vi "Spectral Data Organize TDMS (SubVI).vi"(0 "Measurement Cluster IN":T2, 1 "Data Array IN":dbl[](array[numeric]), 2 "tdms file":refnum<k34>, 3 "error in (no error)":errorcluster, 5 "Shutter":bool, 7 "Ref Lamp Mode":T1(radio), 9 "Collect Background":bool, 10 "Ref Lamp at Flame Loc File":path=path "C:/Users/bedickc/Documents/_MHD/K Spectroscopy (Ocean Optics Spectrometer)/20171005_HR4000_KOptics_Calib/Lamp_At_Flame_Location_ND10Corr_HR4000_LabviewWavelengths.csv", 11 "Take Ref Lamp":bool, 13 "Integration Time (ms)":dbl format="%#_13g", 14 "ON/OFF IN":bool) -> (4 "Measurement Cluster OUT":T2, 6 "tdms file out":refnum<k34>, 8 "error out":errorcluster)   [LabVIEW 2018]
uses:
  Measurement Cluster.ctl
panel:
  in  "Iteration Number":i32
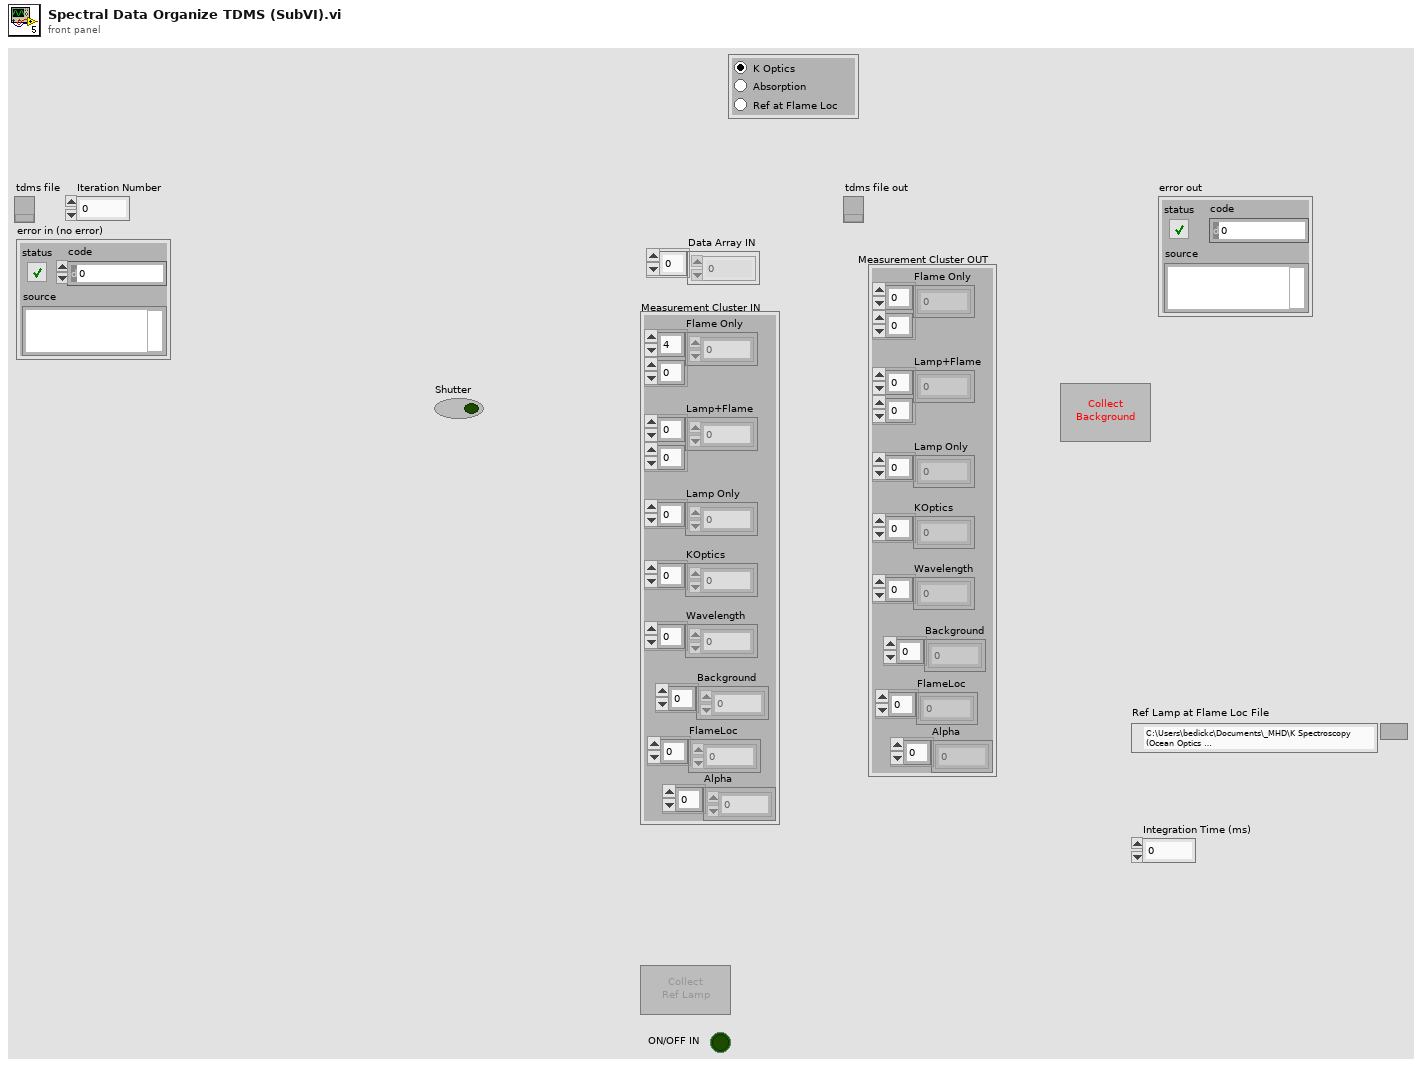
[diagram p1: front panel]
types:
  T1 = enum32{"K Optics", "Absorption", "Ref at Flame Loc"}
  T2 = typedef "Measurement Cluster.ctl" = cluster{"Flame Only":dbl[][], "Lamp+Flame":dbl[][], "Lamp Only":dbl[], "KOptics":dbl[], "Wavelength":dbl[], "Background":dbl[], "FlameLoc":dbl[], "Alpha":dbl[]}
  T3 = enum16{"open", "open or create", "create or replace", "create", "open (read-only)"}
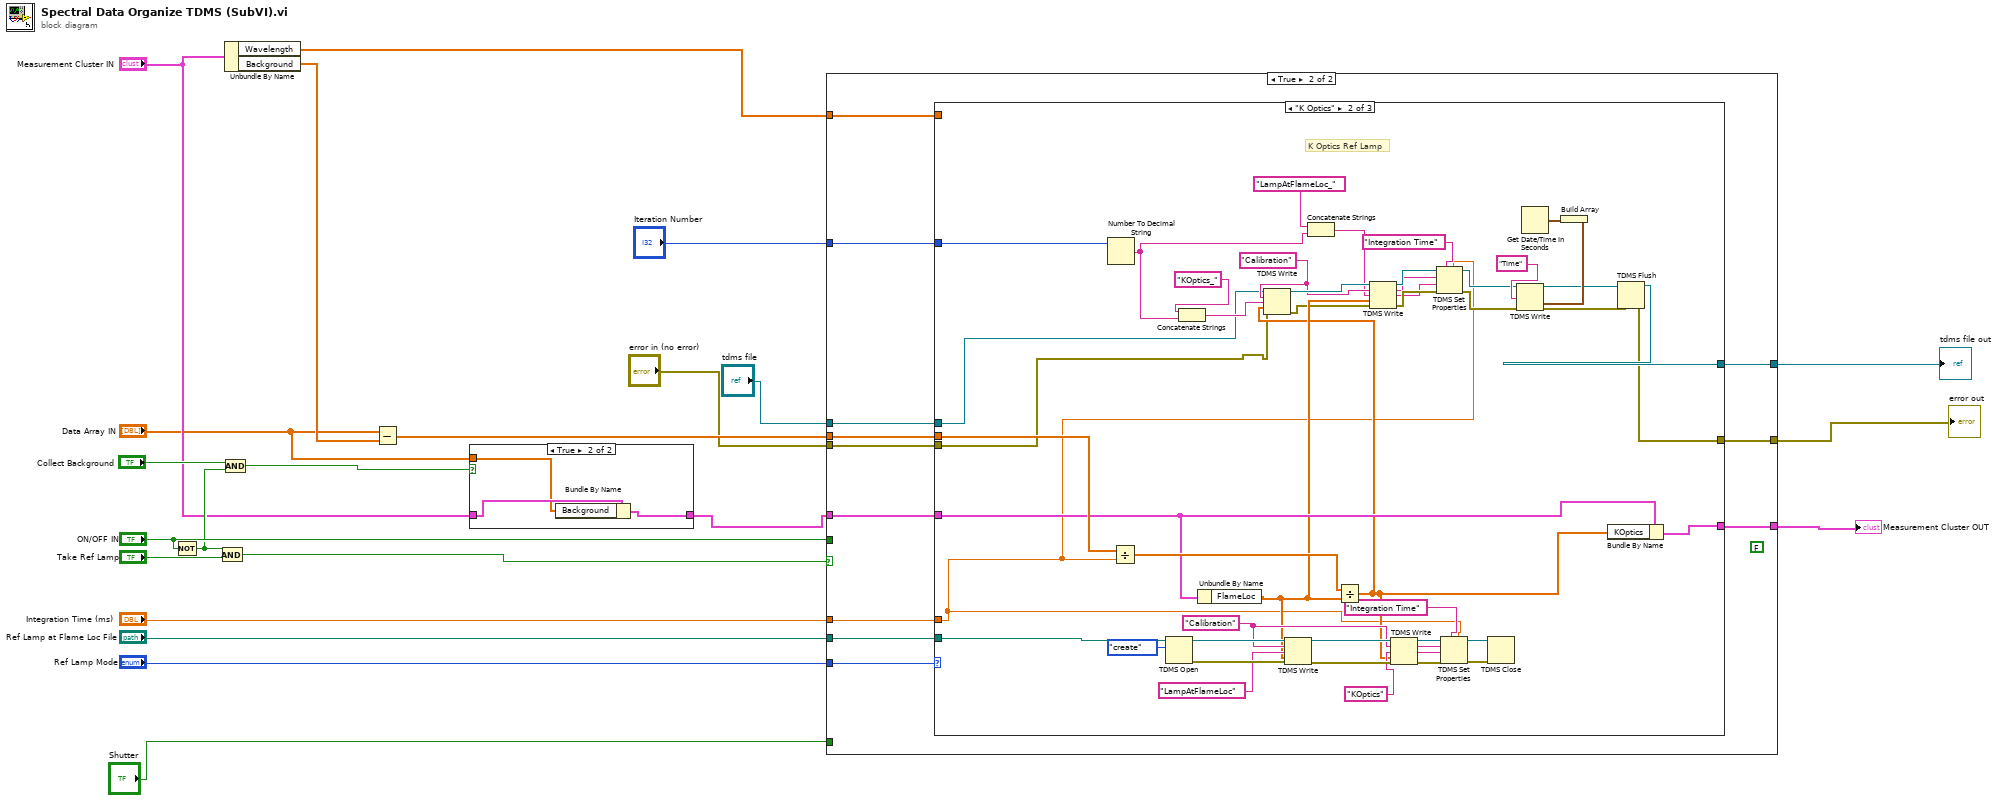
[diagram p0: block diagram]
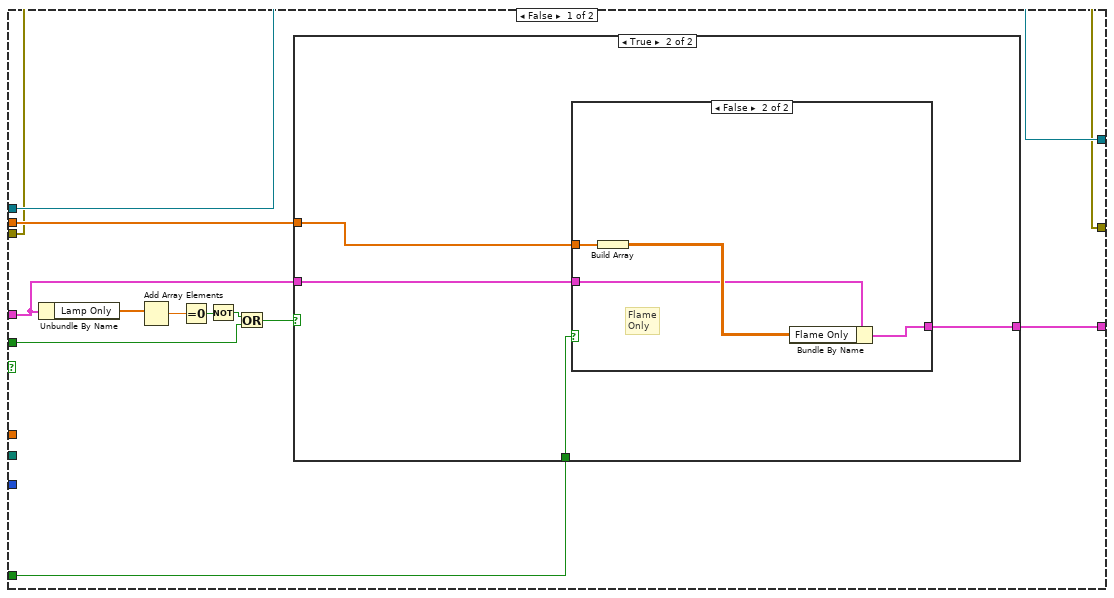
[diagram p2: hidden frame]
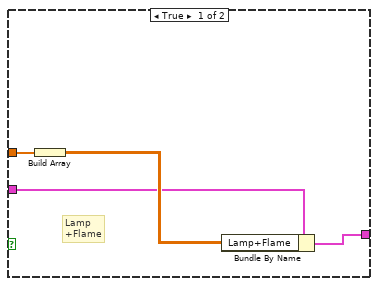
[diagram p4: hidden frame]
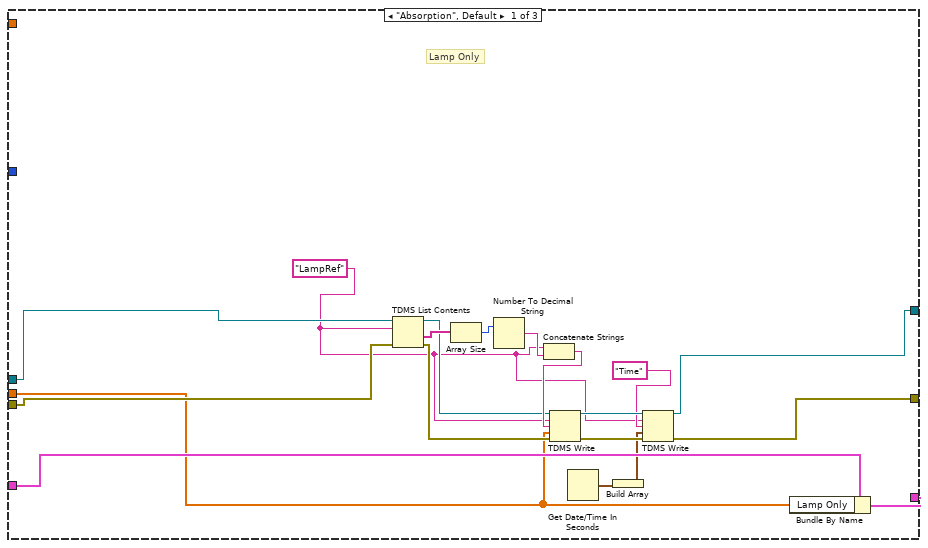
[diagram p5: hidden frame]
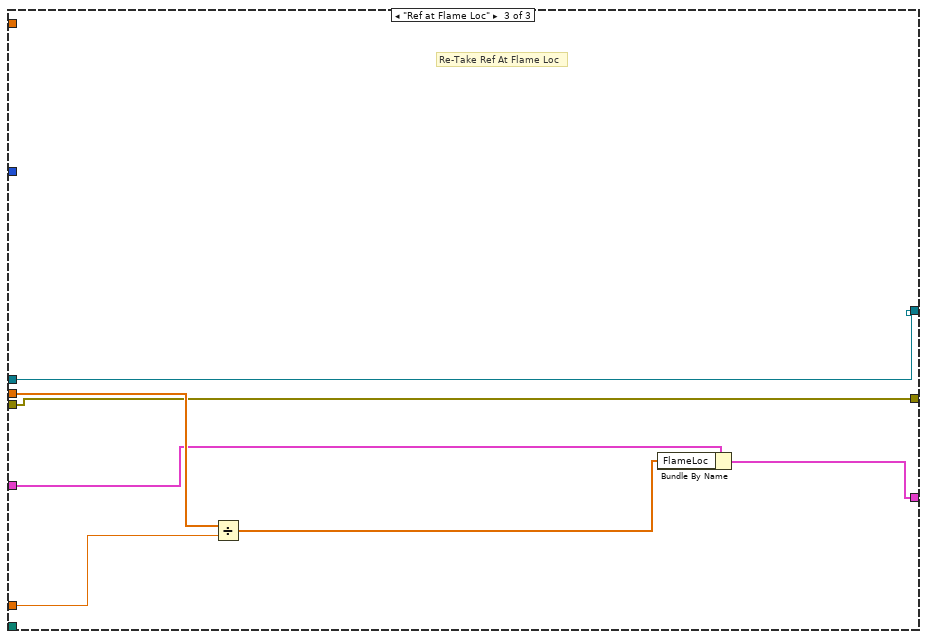
[diagram p6: hidden frame]
diagram:
  n1 = Not(x="ON/OFF IN") -> (.not. x?=w12:bool)
  n2 = Compound Arithmetic op=AND(w12, "Take Ref Lamp") -> (w21:bool)
  n3 = Unbundle By Name("Measurement Cluster IN") -> ("Wavelength"=w19:dbl[], "Background"=w15:dbl[])
  n4 = Compound Arithmetic op=AND("Collect Background", w12) -> (w10:bool)
  n5 = Subtract(x="Data Array IN", y=w15) -> (x-y=w16:dbl[])
  n6 = case shown="True" w10 {
    tunnel: "Measurement Cluster IN" -> [w23 w25]
    tunnel: [w23 w26] -> w6
    tunnel: "Data Array IN" -> [_ w24]
    frame False {
    }
    frame True {
      n7 = Bundle By Name(cluster=w25, "Background"=w24) -> (w26:T2)
    }
  }
  n8 = case shown="True" w21 {
    tunnel: w16 -> [w38 w58]
    tunnel: "ON/OFF IN" -> [w37 _]
    tunnel: "Ref Lamp at Flame Loc File" -> [_ w63]
    tunnel: "Integration Time (ms)" -> [_ w62]
    tunnel: w19 -> [_ w61]
    tunnel: [w34 w60] -> w18
    tunnel: w6 -> [w35 w59]
    tunnel: "Ref Lamp Mode" -> [_ w57]
    tunnel: "Shutter" -> [w31 _]
    tunnel: "tdms file" -> [w28 w56]
    tunnel: "error in (no error)" -> [w27 w55]
    tunnel: [w28 w54] -> w3
    tunnel: [w27 w53] -> w2
    tunnel: "Iteration Number" -> [_ w52]
    frame False {
      n9 = Unbundle By Name(w35) -> ("Lamp Only"=w32:dbl[])
      n10 = Add Array Elements(numeric array=w32) -> (sum=w33:dbl)
      n11 = Equal To 0?(x=w33) -> (x = 0?=w30:bool)
      n12 = Not(x=w30) -> (.not. x?=w29:bool)
      n13 = Or(x=w29, y=w37) -> (x .or. y?=w36:bool)
      n14 = case shown="True" w36 {
        tunnel: w38 -> [_ w43]
        tunnel: w35 -> [w39 w42]
        tunnel: [w39 w41] -> w34
        tunnel: w31 -> [_ w40]
        frame False {
        }
        frame True {
          n15 = case shown="False" w40 {
            tunnel: w43 -> [w47 w51]
            tunnel: w42 -> [w45 w49]
            tunnel: [w44 w48] -> w41
            frame True {
              # "Lamp\n+Flame"
              n16 = Build Array(w47) -> (w46:dbl[][])
              n17 = Bundle By Name(cluster=w45, "Lamp+Flame"=w46) -> (w44:T2)
            }
            frame False {
              # "Flame\nOnly"
              n18 = Build Array(w51) -> (w50:dbl[][])
              n19 = Bundle By Name(cluster=w49, "Flame Only"=w50) -> (w48:T2)
            }
          }
        }
      }
    }
    frame True {
      (unwired) FALSE
      n20 = case shown="\"K Optics\"" w57 {
        tunnel: w63 -> [_ w126 _]
        tunnel: w62 -> [_ w93 w137]
        tunnel: w61 -> [_ _ _]
        tunnel: [w82 w130 w134] -> w60
        tunnel: w59 -> [w81 w127 w135]
        tunnel: w58 -> [w65 w129 w136]
        tunnel: w56 -> [w69 w87 w132]
        tunnel: w55 -> [w68 w86 w131]
        tunnel: [w64 w89 w132] -> w54
        tunnel: [w67 w88 w131] -> w53
        tunnel: w52 -> [_ w106 _]
        frame "Absorption", Default {
          w66 = "LampRef" ("group name in (Untitled)")
          # "Lamp Only"
          n21 = TDMS List Contents(4:w68, 6:w66, 7:w69) -> (0:w75:errorcluster, 1:w80:string[], 3:w76:refnum<k34>)  [unwired: 1 out]
          n22 = Array Size(array=w80) -> (size(s)=w79:i32)
          n23 = Number To Decimal String(number=w79) -> (decimal integer string=w78:string)  [unwired: 1 in]
          n24 = Concatenate Strings(w66, w78) -> (w77:string)
          n25 = TDMS Write(0:w76, 5:w66, 7:w77, 9:w65, 11:w75) -> (4:w74:refnum<k34>, 15:w73:errorcluster)  [unwired: 1 in, 2 out]
          n26 = Get Date/Time In Seconds() -> (seconds since 1Jan1904=w72:timestamp)
          n27 = Build Array(w72) -> (w71:timestamp[])
          n28 = TDMS Write(0:w74, 5:w66, 7:"Time" ("group name in (Untitled)"), 9:w71, 11:w73) -> (4:w64:refnum<k34>, 15:w67:errorcluster)  [unwired: 1 in, 2 out]
          n29 = Bundle By Name(cluster=w81, "Lamp Only"=w65) -> (w82:T2)
        }
        frame "K Optics" {
          w108 = "Calibration" ("group name in (Untitled)")
          w119 = "Calibration" ("group name in (Untitled)")
          # "K Optics Ref Lamp"
          n30 = Number To Decimal String(number=w106) -> (decimal integer string=w103:string)  [unwired: 1 in]
          n31 = Divide(x=w129, y=w93) -> (x/y=w128:dbl[])
          n32 = TDMS Open(10:T3."create" ("operation (0:open)"), 11:w126) -> (0:w124:errorcluster, 3:w125:refnum<k34>)  [unwired: 5 in]
          n33 = Concatenate Strings("KOptics_" ("group name in (Untitled)"), w103) -> (w92:string)
          n34 = Unbundle By Name(w127) -> ("FlameLoc"=w101:dbl[])
          n35 = TDMS Write(0:w125, 5:w119, 7:"LampAtFlameLoc" ("group name in (Untitled)"), 9:w101, 11:w124) -> (4:w121:refnum<k34>, 15:w120:errorcluster)  [unwired: 1 in, 2 out]
          n36 = Concatenate Strings("LampAtFlameLoc_" ("group name in (Untitled)"), w103) -> (w102:string)
          n37 = Divide(x=w128, y=w101) -> (x/y=w100:dbl[])
          n38 = TDMS Write(0:w87, 5:w108, 7:w92, 9:w100, 11:w86) -> (4:w109:refnum<k34>, 15:w85:errorcluster)  [unwired: 1 in, 2 out]
          n39 = TDMS Write(0:w109, 5:w108, 7:w102, 9:w101, 11:w85) -> (4:w98:refnum<k34>, 6:w84:string, 8:w83:string, 15:w97:errorcluster)  [unwired: 1 in]
          n40 = TDMS Write(0:w121, 5:w119, 7:"KOptics" ("group name in (Untitled)"), 9:w100, 11:w120) -> (4:w114:refnum<k34>, 6:w115:string, 8:w116:string, 15:w117:errorcluster)  [unwired: 1 in]
          n41 = TDMS Set Properties(5:w93, 7:"Integration Time" ("group name in (Untitled)"), 8:w97, 9:w83, 10:w84, 11:w98) -> (0:w95:errorcluster, 3:w96:refnum<k34>)  [unwired: 2 out]
          n42 = TDMS Set Properties(5:w93, 7:"Integration Time" ("group name in (Untitled)"), 8:w117, 9:w116, 10:w115, 11:w114) -> (0:w113:errorcluster, 3:w112:refnum<k34>)  [unwired: 2 out]
          n43 = TDMS Close(8:w113, 11:w112) -> ()  [unwired: 2 out]
          n44 = Get Date/Time In Seconds() -> (seconds since 1Jan1904=w111:timestamp)
          n45 = Build Array(w111) -> (w107:timestamp[])
          n46 = TDMS Write(0:w96, 7:"Time" ("group name in (Untitled)"), 9:w107, 11:w95) -> (4:w91:refnum<k34>, 15:w90:errorcluster)  [unwired: 2 in, 2 out]
          n47 = Bundle By Name(cluster=w127, "KOptics"=w100) -> (w130:T2)
          n48 = TDMS Flush(4:w90, 7:w91) -> (0:w88:errorcluster, 3:w89:refnum<k34>)
        }
        frame "Ref at Flame Loc" {
          # "Re-Take Ref At Flame Loc"
          n49 = Divide(x=w136, y=w137) -> (x/y=w133:dbl[])
          n50 = Bundle By Name(cluster=w135, "FlameLoc"=w133) -> (w134:T2)
        }
      }
    }
  }
  "Measurement Cluster OUT" <- w18
  "tdms file out" <- w3
  "error out" <- w2
